vi "VariantArrayAccessMulti.vi"(8 "error in (no error)":errorcluster, 10 "Indices":i32[](array[numeric]), 11 "Array":variant) -> (0 "error out":errorcluster, 1 "rest":string, 2 "value":variant, 3 "prepend":string, 5 "array size":u32[](array[numeric]), 7 "type string":i16[](array[numeric]))   [LabVIEW 2021]
uses:
  <vilib>/Utility/Data Type/NI_Data Type.lvlib
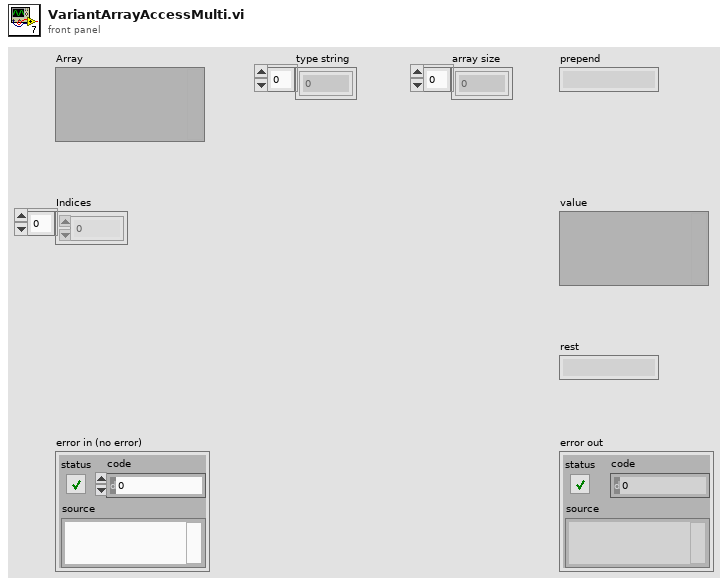
[diagram p1: front panel]
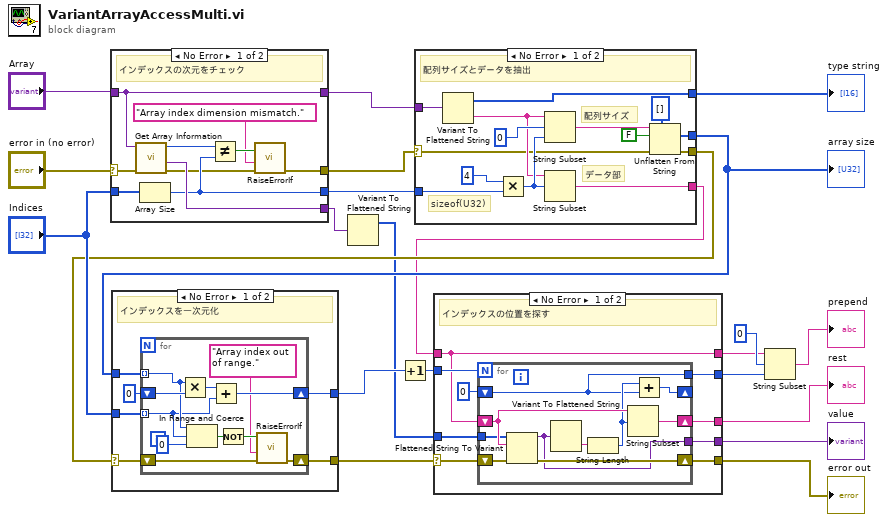
[diagram p0: block diagram]
diagram:
  n1 = case shown="No Error" "error in (no error)" {
    selector: "error in (no error)" -> [w24 w33]
    tunnel: "Array" -> [w23 _]
    tunnel: "Indices" -> [w32 _]
    tunnel: [w31 _] -> w20
    tunnel: [w29 _] -> w19
    tunnel: [w27 w33] -> w8
    tunnel: [w23 _] -> w15
    frame No Error {
      # "インデックスの次元をチェック"
      n2 = call <vilib>:"Get Array Information.vi"("error in (no error)"=w24, "variant"=w23) -> ("error out"=w28:errorcluster, "array element data type"=w31:variant, "number of dimensions"=w30:i32)  [unwired: 6 in, 1 out]
      n3 = Array Size(array=w32) -> (size(s)=w29:i32)
      n4 = Not Equal?(x=w30, y=w29) -> (x != y?=w26:bool)
      n5 = call "RaiseErrorIf.vi"("error in (no error)"=w28, "error message"="Array index dimension mismatch.", "error? (true)"=w26) -> ("error out"=w27:errorcluster)  [unwired: 8 in]
    }
    frame Error {
    }
  }
  n6 = Variant To Flattened String(Variant=w20) -> (1:w2:i16[])  [unwired: 1 out]
  n7 = case shown="No Error" w8 {
    selector: w8 -> [w34 w48]
    tunnel: w19 -> [w47 _]
    tunnel: [w41 _] -> w17
    tunnel: [w39 w48] -> w7
    tunnel: w15 -> [w37 _]
    tunnel: [w36 _] -> w14
    tunnel: [w35 _] -> w3
    frame No Error {
      # "sizeof(U32)"
      # "データ部"
      # "配列サイズ"
      # "配列サイズとデータを抽出"
      n8 = Variant To Flattened String(Variant=w37) -> (data string=w44:string, 1:w36:i16[])
      n9 = Multiply(x=4, y=w47) -> (x*y=w46:i32)
      n10 = String Subset(string=w44, offset (0)=0, length (rest)=w46) -> (substring=w40:string)
      n11 = String Subset(string=w44, offset (0)=w46) -> (substring=w35:string)  [unwired: 1 in]
      n12 = Unflatten From String(type=u32[] [], binary string=w40, data includes array or string size? (T)=FALSE, error in (no error)=w34) -> (value=w41:u32[], error out=w39:errorcluster)  [unwired: 1 in, 1 out]
    }
    frame Error {
    }
  }
  "type string" <- w14
  "array size" <- w17
  n13 = case shown="No Error" w7 {
    selector: w7 -> [w49 w66]
    tunnel: "Indices" -> [w54 _]
    tunnel: w17 -> [w52 _]
    tunnel: [w51 w66] -> w6
    tunnel: [w50 _] -> w13
    frame No Error {
      # "インデックスを一次元化"
      n14 = for {
        tunnel: w54 -> [w60] mode=indexing
        shift-right: [w63] -> w50
        shift-left: 0 -> [w65]
        tunnel: w52 -> [w62] mode=indexing
        shift-right: [w56] -> w51
        shift-left: w49 -> [w57]
        n15 = Multiply(x=w62, y=w65) -> (x*y=w64:u32)
        n16 = In Range and Coerce(upper limit=w62, x=w60, lower limit=u32 0) -> (In Range?=w59:bool)  [unwired: 1 out]
        n17 = Add(x=w64, y=w60) -> (x+y=w63:u32)
        n18 = Not(x=w59) -> (.not. x?=w58:bool)
        n19 = call "RaiseErrorIf.vi"("error in (no error)"=w57, "error message"="Array index out of range.", "error? (true)"=w58) -> ("error out"=w56:errorcluster)  [unwired: 8 in]
      }
    }
    frame Error {
    }
  }
  n20 = Increment(x=w13) -> (x+1=w1:u32)
  n21 = case shown="No Error" w6 {
    selector: w6 -> [w70 w86]
    tunnel: [w75 w86] -> w18
    tunnel: w2 -> [w74 _]
    tunnel: w1 -> [w73 _]
    tunnel: [w67 _] -> w12
    tunnel: [w71 _] -> w9
    tunnel: w3 -> [w68 _]
    tunnel: [w69 _] -> w5
    tunnel: [w68 _] -> w4
    frame No Error {
      # "インデックスの位置を探す"
      n22 = for {
        N: w73 -> [_]
        shift-right: [w85] -> w69
        shift-left: w68 -> [w84]
        shift-right: [w80] -> w75
        shift-left: w70 -> [w82]
        tunnel: w74 -> [w81]
        shift-right: [w79] -> _
        shift-left: u32 0 -> [w76]
        tunnel: [w77] -> w71
        tunnel: [w76] -> w67
        n23 = Flattened String To Variant(4:w82, 6:w84, 7:w81) -> (0:w80:errorcluster, 3:w77:variant)
        n24 = Variant To Flattened String(Variant=w77) -> (data string=w83:string)  [unwired: 1 out]
        n25 = String Length(string=w83) -> (length=w78:i32)
        n26 = String Subset(string=w84, offset (0)=w78) -> (substring=w85:string)  [unwired: 1 in]
        n27 = Add(x=w78, y=w76) -> (x+y=w79:u32)
      }
    }
    frame Error {
    }
  }
  "error out" <- w18
  "rest" <- w5
  "value" <- w9
  n28 = String Subset(string=w4, offset (0)=0, length (rest)=w12) -> (substring=→"prepend":string)
